vi "Handle Errors.vi"(8 "error in (no error)":errorcluster, 10 "Location":string, 11 "Helper Loop In":refnum<class "Helper Loop.lvclass">) -> (0 "error out":errorcluster, 3 "Helper Loop Out":refnum<class "Helper Loop.lvclass">)   [LabVIEW 2020, in "Helper Loop.lvclass"]
doc: "The implementation of this VI defines how errors are handled."
uses:
  Helper Loop.lvclass
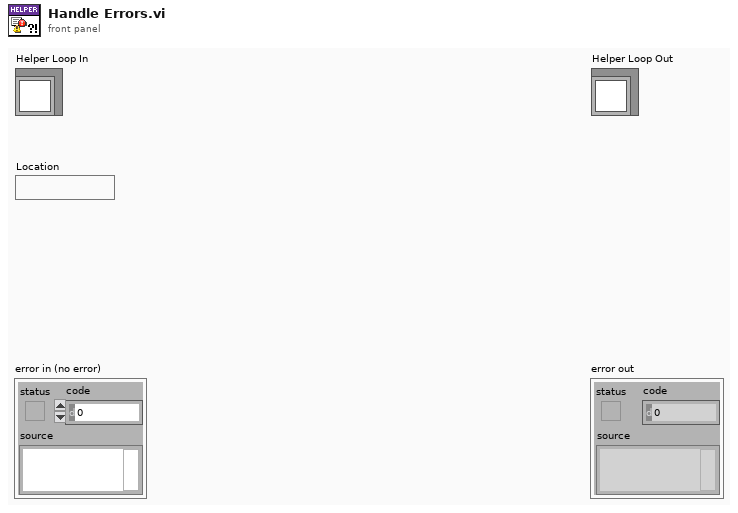
[diagram p1: front panel]
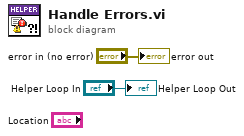
[diagram p0: block diagram]
diagram:
  "error out" <- "error in (no error)"
  "Helper Loop Out" <- "Helper Loop In"
